vi "Add Engine Simulation Toolkit Custom Device.vi"(8 "error in (no error)":errorcluster, 10 "Settings":T1={"Name"="", "Execution priority"=enum."Medium", "Rate decimation"=1, "CPU"=-2} {"Rate decimation" min=1}, 11 "Target in":refnum<k24>) -> (0 "error out":errorcluster, 2 "EST Custom Device":refnum<k24>, 3 "Target out":refnum<k24>)   [LabVIEW 2015, in "Engine Simulation Toolkit Scripting API.lvlib"]
uses:
  Engine Simulation Toolkit Scripting API.lvlib
  NationalInstruments.VeriStand.SystemDefinitionAPI
  Engine Simulation Toolkit Custom Device Settings.ctl
  Shared/Constants and GUIDs.vi
  Shared/Properties.vi
  <vilib>/NI Veristand/Custom Device API/Set Item Property (I32).vi
  Shared/Engine Simulation Toolkit Shared.lvlib
  <vilib>/NI VeriStand/Custom Device API/Custom Device API.lvlib
  System Explorer/Engine Simulation Toolkit System Explorer.lvlib
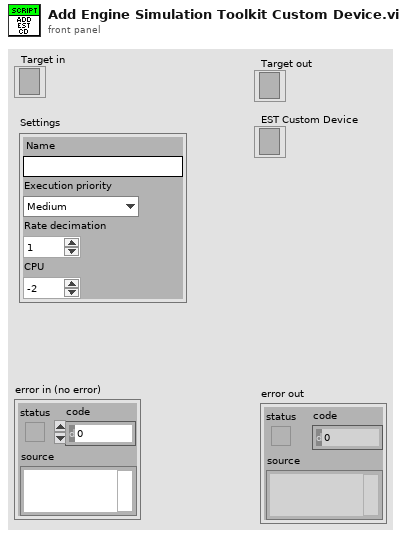
[diagram p1: front panel]
types:
  T1 = typedef "Engine Simulation Toolkit Scripting API.lvlib/Engine Simulation Toolkit Custom Device Settings.ctl" = cluster{"Name":string, "Execution priority":enum16{"Low", "Medium", "High"}, "Rate decimation":i32, "CPU":i32}
  T2 = typedef "Custom Device API.lvlib/Custom Device Item Ref.ctl" = u64
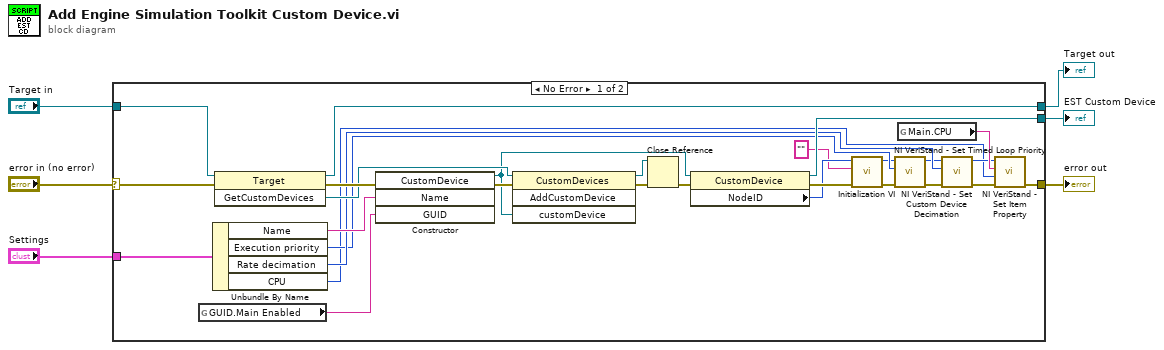
[diagram p0: block diagram]
diagram:
  n1 = case shown="No Error" "error in (no error)" {
    selector: "error in (no error)" -> [w34 w36]
    tunnel: [w12 w36] -> w6
    tunnel: "Target in" -> [w33 w35]
    tunnel: [w26 w35] -> w3
    tunnel: "Settings" -> [w32 _]
    tunnel: [w21 _] -> w1
    frame No Error {
      n2 = global read "Constants and GUIDs.vi" "GUID.Main Enabled"() -> (w29:string)
      n3 = Unbundle By Name(w32) -> ("Name"=w30:string, "Execution priority"=w18:enum16{"Low", "Medium", "High"}, "Rate decimation"=w20:i32, "CPU"=w15:i32)
      n4 = invoke class="Target" method="GetCustomDevices"(reference=w33, error in=w34) -> (reference out=w26:refnum<k24>, error out=w31:errorcluster, "GetCustomDevices"=w28:refnum<k24>)  [unwired: 1 in]
      n5 = constructor class="CustomDevice"(error in=w31, "Name"=w30, "GUID"=w29) -> (reference out=w23:refnum<k24>, error out=w27:errorcluster)  [unwired: 2 in, 3 out]
      n6 = invoke class="CustomDevices" method="AddCustomDevice"(reference=w28, error in=w27, "customDevice"=w23) -> (reference out=w25:refnum<k24>, error out=w24:errorcluster)  [unwired: 1 in, 2 out]
      n7 = Close Reference(reference=w25, error in (no error)=w24) -> (error out=w22:errorcluster)
      n8 = property class="CustomDevice"(reference=w23, error in=w22) -> (reference out=w21:refnum<k24>, error out=w10:errorcluster, "NodeID"=w9:u64)
      n9 = call "Initialization VI.vi"("error in (no error)"=w10, "Custom XML"="", "Device Item Ref in"=w9) -> ("error out"=w11:errorcluster, "Device Item Ref out"=w8:T2)  [unwired: 7 in]
      n10 = call <vilib>:"NI VeriStand - Set Timed Loop Priority.vi"("error in (no error)"=w11, "Priority"=w18, "Device Ref in"=w8) -> ("error out"=w13:errorcluster, "Device Ref out"=w19:T2)  [unwired: 7 in]
      n11 = global read "Properties.vi" "Main.CPU"() -> (w17:string)
      n12 = call <vilib>:"NI VeriStand - Set Custom Device Decimation.vi"("error in (no error)"=w13, "Decimation"=w20, "Device Ref in"=w19) -> ("error out"=w14:errorcluster, "Device Ref out"=w16:T2)  [unwired: 7 in]
      n13 = call-poly <vilib>:"NI VeriStand - Set Item Property.vi"("error in (no error)"=w14, "Value"=w15, "Property Name"=w17, "Item Ref in"=w16) -> ("error out"=w12:errorcluster)  [unwired: 5 in, 2 out]
    }
    frame Error {
    }
  }
  "Target out" <- w3
  "error out" <- w6
  "EST Custom Device" <- w1
